vi "Disconnect PV.vi"(8 "error in (no error)":errorcluster, 10 "PV URL":string, 11 "CS++DIMMonitor in":refnum<class "CS++DIMMonitor.lvclass">) -> (0 "error out":errorcluster, 3 "CS++DIMMonitor out":refnum<class "CS++DIMMonitor.lvclass">)   [LabVIEW 2014, in "CS++DIMMonitor.lvlib" / "CS++DIMMonitor.lvclass"]
doc: "Close connection to process variable."
uses:
  CS++DIMMonitor.lvclass
  DimLVEvent/LVDimInterface/LVDimInterface.lvlib
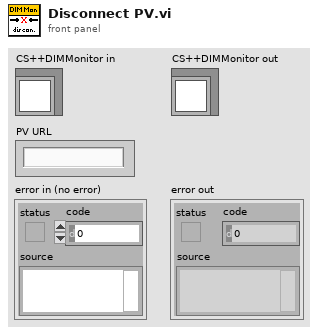
[diagram p1: front panel]
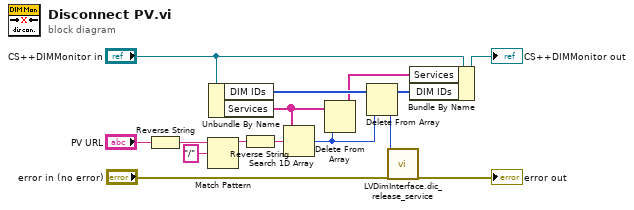
[diagram p0: block diagram]
diagram:
  n1 = Reverse String(1:"PV URL") -> (0:w14:string)
  n2 = Match Pattern(string=w14, regular expression="/" ("search string/char (-)")) -> (before substring=w13:string)  [unwired: 1 in, 3 out]
  n3 = Unbundle By Name("CS++DIMMonitor in") -> ("DIM IDs"=w10:i32[], "Services"=w9:string[])
  n4 = Reverse String(1:w13) -> (0:w11:string)
  n5 = Search 1D Array(1D array=w9, element=w11) -> (index of element=w8:i32)  [unwired: 1 in]
  n6 = Delete From Array(array=w9, index=w8) -> (array with subset deleted=w3:string[])  [unwired: 1 in, 1 out]
  n7 = Delete From Array(array=w10, index=w8) -> (deleted portion=w4:i32, array with subset deleted=w5:i32[])  [unwired: 1 in]
  n8 = call "LVDimInterface.dic_release_service.vi"("callBackID"=w4, "error in (no error)"="error in (no error)") -> ("error out"=→"error out":errorcluster)  [unwired: 17 in]
  n9 = Bundle By Name(cluster="CS++DIMMonitor in", "Services"=w3, "DIM IDs"=w5) -> (→"CS++DIMMonitor out":refnum<class "CS++DIMMonitor.lvclass">)
